vi "CALibration.vi"(8 "Error in (no error)":errorcluster, 10 "Function":T1(ring), 11 "VISA resource":refnum<visa-resource-name>) -> (0 "Error out":errorcluster, 2 "State":string, 3 "Dup VISA resource":refnum<visa-resource-name>)   [LabVIEW 2010]
doc: "Copyright (c) 2012 Metrolab Technology SA, Plan-les-Ouates, Geneva, Switzerland\nCollects all functions dealing with the device calibration."
panel:
  # "CALibration"
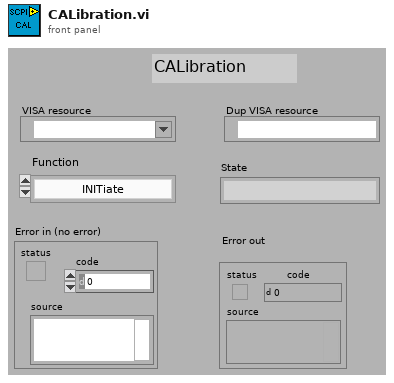
[diagram p1: front panel]
types:
  T1 = enum16{"INITiate", "ZERO", "STATe query", "STATe ON", "STATe OFF"}
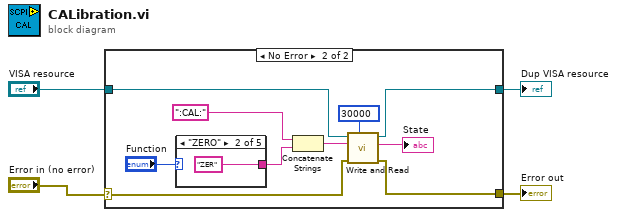
[diagram p0: block diagram]
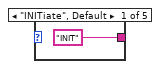
[diagram p3: hidden frame]
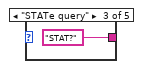
[diagram p4: hidden frame]
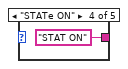
[diagram p5: hidden frame]
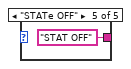
[diagram p6: hidden frame]
diagram:
  n1 = case shown="No Error" "Error in (no error)" {
    selector: "Error in (no error)" -> [w6 w14]
    tunnel: [w6 w13] -> w4
    tunnel: [w5 w8] -> w2
    tunnel: "VISA resource" -> [w5 w7]
    frame Error {
    }
    frame No Error {
      n2 = case shown="\"ZERO\"" "Function" {
        tunnel: ["INIT" "ZER" "STAT?" "STAT ON" "STAT OFF"] -> w9
        frame "INITiate", Default {
        }
        frame "ZERO" {
        }
        frame "STATe query" {
        }
        frame "STATe ON" {
        }
        frame "STATe OFF" {
        }
      }
      n3 = Concatenate Strings(":CAL:", w9) -> (w15:string)
      n4 = call "Write and Read.vi"("Timeout (ms)"=u32 30000, "Error in (no error)"=w14, "Command"=w15, "VISA resource"=w7) -> ("Error out"=w13:errorcluster, "Response"=→"State":string, "Dup VISA resource"=w8:refnum<visa-resource-name>)  [unwired: 3 in, 2 out]
    }
  }
  "Error out" <- w4
  "Dup VISA resource" <- w2
